vi "THFL1dll.vi"(8 "error in (no error)":errorcluster, 11 "Inputs":T2) -> (0 "error out":errorcluster, 3 "Outputs":T1)   [LabVIEW 2016]
uses:
  REFPROP.DLL
panel:
  # "REFPROP-THFL1dll.vi"
  # "void  TEFL1dll(double *t, double *h, double *z, double *dmin, double dmax, double d, int32_t *ierr, CStr herr, int32_t herr_length);"
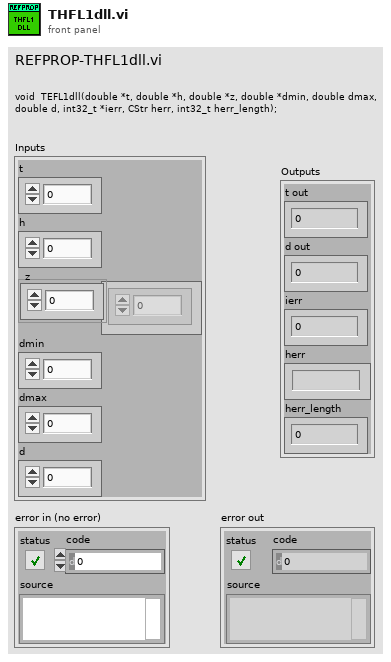
[diagram p1: front panel]
types:
  T1 = cluster{"t out":dbl, "d out":dbl, "ierr":i32, "herr":string, "herr_length":i32}
  T2 = cluster{"t":dbl, "h":dbl, "z":dbl[], "dmin":dbl, "dmax":dbl, "d":dbl}
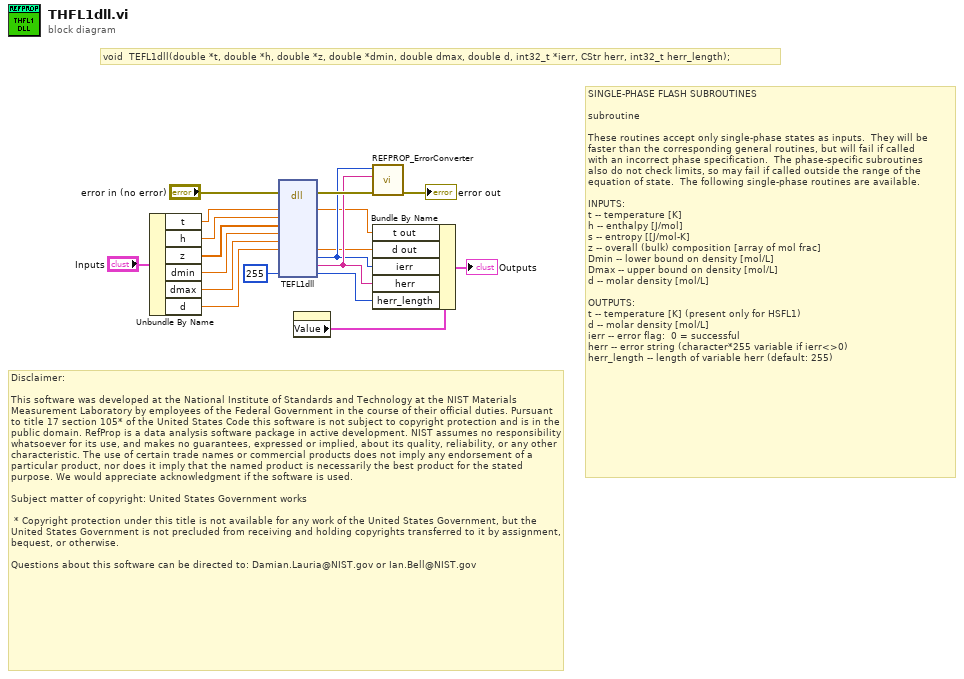
[diagram p0: block diagram]
diagram:
  # "Disclaimer:\n\nThis software was developed at the National Institute of Standards and Technology at the NIST Materials Measurement Laboratory by employees of the Federal Government in the course of their official duties. Pursuant to title 17 section 105* of the United States Code this software is not subject to copyright protection and is in the public domain. RefProp is a data analysis software package in active development. NIST assumes no responsibility whatsoever for its use, and makes no guarantees, expressed or implied, about its quality, reliability, or any other characteristic. The use of certain trade names or commercial products does not imply any endorsement of a particular product, nor does it imply that the named product is necessarily the best product for the stated purpose. We would appreciate acknowledgment if the software is used.\n \nSubject matter of copyright: United States Government works\n  \n * Copyright protection under this title is not available for any work of the United States Government, but the United States Government is not precluded from receiving and holding copyrights transferred to it by assignment, bequest, or otherwise.\n\nQuestions about this software can be directed to: Damian.Lauria@NIST.gov or Ian.Bell@NIST.gov"
  # "void  TEFL1dll(double *t, double *h, double *z, double *dmin, double dmax, double d, int32_t *ierr, CStr herr, int32_t herr_length);"
  # "SINGLE-PHASE FLASH SUBROUTINES\n\nsubroutine \n\nThese routines accept only single-phase states as inputs.  They will be\nfaster than the corresponding general routines, but will fail if called\nwith an incorrect phase specification.  The phase-specific subroutines\nalso do not check limits, so may fail if called outside the range of the\nequation of state.  The following single-phase routines are available.\n\nINPUTS: \nt -- temperature [K]\nh -- enthalpy [J/mol]\ns -- entropy [[J/mol-K]\nz -- overall (bulk) composition [array of mol frac]\nDmin -- lower bound on density [mol/L]\nDmax -- upper bound on density [mol/L]\nd -- molar density [mol/L]\n\nOUTPUTS:\nt -- temperature [K] (present only for HSFL1)\nd -- molar density [mol/L]\nierr -- error flag:  0 = successful\nherr -- error string (character*255 variable if ierr<>0)\nherr_length -- length of variable herr (default: 255)"
  n1 = Unbundle By Name("Inputs") -> ("t"=w6:dbl, "h"=w7:dbl, "z"=w8:dbl[], "dmin"=w9:dbl, "dmax"=w10:dbl, "d"=w11:dbl)
  n2 = dll-call lib="S:/009 - Testing/02 - Performance Testing/REFPROP/REFPROP.*" fn="TEFL1dll"(error in="error in (no error)", "t"=w6, "h"=w7, "z"=w8, "dmin"=w9, "dmax"=w10, "d"=w11, "herr_length"=255) -> (error out=w15:errorcluster, "t"=w1:dbl, "d"=w2:dbl, "ierr"=w3:i32, "herr"=w4:string, "herr_length"=w5:i32)  [unwired: 9 in, 1 out]
  n3 = property on="Outputs" class="Clust (strict)"() -> ("Value"=w16:T1)  [unwired: 2 in, 2 out]
  n4 = call "REFPROP_ErrorConverter.vi"("error in (no error)"=w15, "Error Message"=w4, "Error Code"=w3) -> ("error out"=→"error out":errorcluster)  [unwired: 8 in]
  n5 = Bundle By Name(cluster=w16, "t out"=w1, "d out"=w2, "ierr"=w3, "herr"=w4, "herr_length"=w5) -> (→"Outputs":T1)
